vi "dialogue.vi"(0 "Cancel":bool, 1 "OK":bool, 2 "Author":string, 10 "HDF5 Save":path[](array[path])=[path "", path ""], 11 "RID":string) -> ()   [LabVIEW 2015, in "oskar_tools.lvlib"]
uses:
  oskar_tools.lvlib
  <vilib>/UPVI/lvhdf5/attribute.llb/Simple H5Awrite (Variant).vi
  <vilib>/UPVI/lvhdf5/attribute.llb/LVH5A Operation.ctl
  <vilib>/UPVI/lvhdf5/attribute.llb/Simple H5Awrite.xnode
  <vilib>/UPVI/lvhdf5/library.llb/HDF5 Ref.ctl
panel:
  in  "Description":string
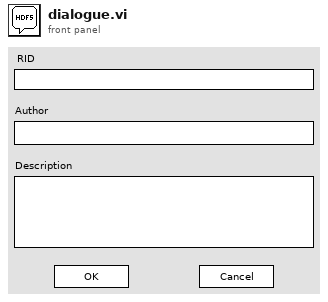
[diagram p1: front panel]
types:
  T1 = typedef "Semaphore RefNum" = refnum<k1>
  T2 = typedef "HDF5 Ref.ctl" = refnum<k1>
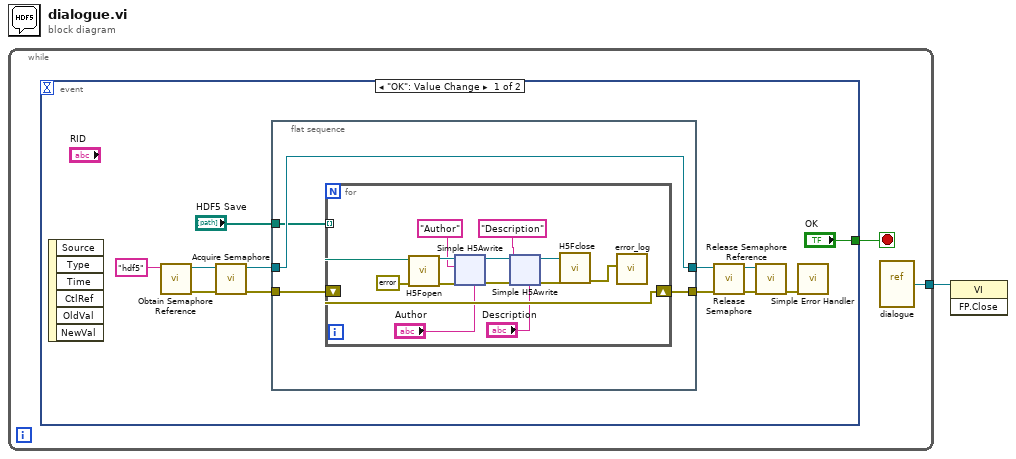
[diagram p0: block diagram]
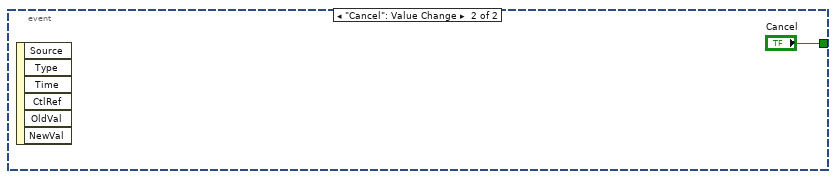
[diagram p2: hidden frame]
diagram:
  n1 = while {
    tunnel: [w2] -> w1
    stop <- w3 stop-if-true
    n2 = event shown="[0] \"OK\": Value Change" {
      selector: _ -> [_ _]
      dyn-events: _ -> [_ _]
      timeout: _ -> [_ _]
      tunnel: ["OK" "Cancel"] -> w3
      event "OK": Value Change {
        n3 = event-data() -> ()  [unwired: 1 in, 6 out]
        n4 = call <vilib>:"Obtain Semaphore Reference.vi"("name (unnamed)"="hdf5") -> ("error out"=w13:errorcluster, "semaphore"=w14:T1)  [unwired: 4 in, 1 out]
        n5 = call <vilib>:"Acquire Semaphore.vi"("error in (no error)"=w13, "semaphore"=w14) -> ("error out"=w7:errorcluster, "semaphore out"=w8:T1)  [unwired: 3 in, 1 out]
        n6 = flat-sequence {
          tunnel: [w19] -> w9
          tunnel: w8 -> [w19]
          tunnel: w7 -> [w17]
          tunnel: "HDF5 Save" -> [w18]
          tunnel: [w16] -> w5
          frame #0 {
            n7 = for {
              tunnel: w18 -> [w31] mode=indexing
              shift-right: [w33] -> w16
              shift-left: w17 -> [w33]
              n8 = call <vilib>:"H5Fopen.vi"("error in (no error)"=errorcluster {"status"=FALSE, "code"=0, "source"=""}, "path"=w31) -> ("error out"=w25:errorcluster, "HDF5 Ref out"=w24:T2)  [unwired: 6 in]
              n9 = xnode "Simple H5Awrite"("HDF5 Ref"=w24, "Name"="Author" ("attrib name"), "error in (no error)"=w25, "Value"="Author") -> ("HDF5 Ref out"=w26:T2, "error out"=w29:errorcluster)  [unwired: 1 in]
              n10 = xnode "Simple H5Awrite"("HDF5 Ref"=w26, "Name"="Description" ("attrib name"), "error in (no error)"=w29, "Value"="Description") -> ("HDF5 Ref out"=w27:T2, "error out"=w28:errorcluster)  [unwired: 1 in]
              n11 = call <vilib>:"H5Fclose.vi"("error in (no error)"=w28, "HDF5 Ref"=w27) -> ("error out"=w30:errorcluster)  [unwired: 7 in]
              n12 = call "error_log.vi"("error"=w30) -> ()  [unwired: 10 in]
            }
          }
        }
        n13 = call <vilib>:"Release Semaphore.vi"("error in (no error)"=w5, "semaphore"=w9) -> ("error out"=w11:errorcluster, "semaphore out"=w10:T1)  [unwired: 4 in]
        n14 = call <vilib>:"Release Semaphore Reference.vi"("error in (no error)"=w11, "semaphore"=w10) -> ("error out"=w4:errorcluster)  [unwired: 8 in, 1 out]
        n15 = call <vilib>:"Simple Error Handler.vi"("error in (no error)"=w4) -> ()  [unwired: 4 in, 5 out]
      }
      event "Cancel": Value Change {
        n16 = event-data() -> ()  [unwired: 1 in, 6 out]
      }
    }
    n17 = vi-ref "dialogue.vi"() -> (w2:refnum<vi>)
  }
  n18 = invoke class="VI" method="FP.Close"(reference=w1) -> ()  [unwired: 2 in, 3 out]
